vi "DebianFile.vi"(8 "error in (no error)":errorcluster, 11 "Package Builder in":refnum<class "Package Builder.lvclass">) -> (0 "error out":errorcluster, 3 "Package Builder out":refnum<class "Package Builder.lvclass">)   [LabVIEW 2020, in "Package Builder.lvclass"]
uses:
  Package Builder.lvclass
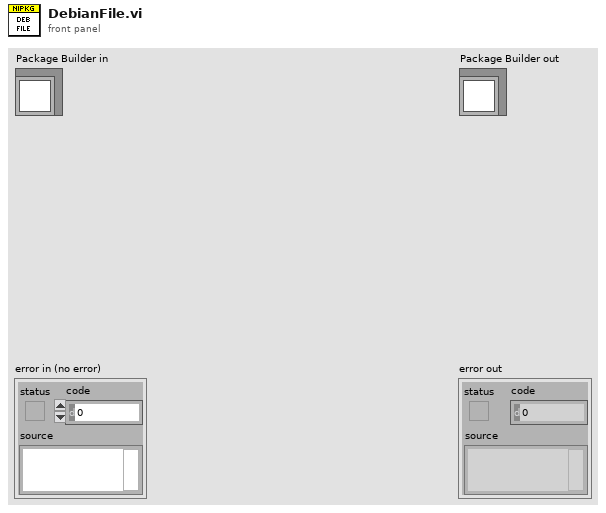
[diagram p1: front panel]
types:
  T1 = enum16{"open", "replace", "create", "open or create", "replace or create", "replace or create with confirmation"}
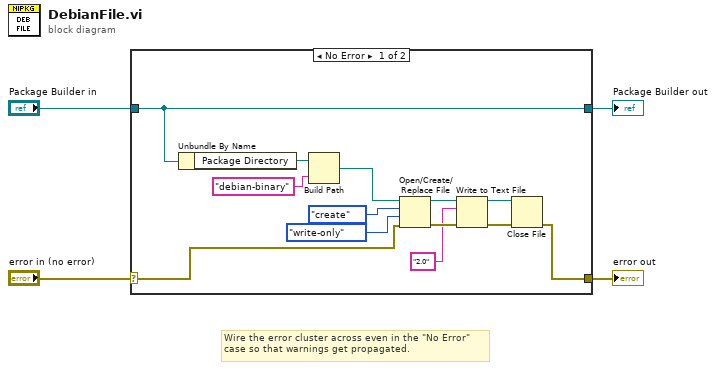
[diagram p0: block diagram]
diagram:
  # "Wire the error cluster across even in the \"No Error\"\ncase so that warnings get propagated."
  n1 = case shown="No Error" "error in (no error)" {
    selector: "error in (no error)" -> [w6 w19]
    tunnel: [w5 w19] -> w3
    tunnel: [w8 w18] -> w1
    tunnel: "Package Builder in" -> [w8 w18]
    frame No Error {
      n2 = Unbundle By Name(w8) -> ("Package Directory"=w7:path)
      n3 = Build Path(base path=w7, name or relative path="debian-binary" ("time format string (%c)")) -> (appended path=w10:path)
      n4 = Open/Create/Replace File(file path (use dialog)=w10, error in=w6, operation (0:open)=T1."create", access (0:read/write)=enum16{"read/write", "read-only", "write-only"}."write-only") -> (refnum out=w15:refnum<file>, error out=w14:errorcluster)  [unwired: 2 in, 1 out]
      n5 = Write to Text File(file (use dialog)=w15, text="2.0", error in=w14) -> (refnum out=w16:refnum<file>, error out=w17:errorcluster)  [unwired: 1 in, 1 out]
      n6 = Close File(refnum=w16, error in=w17) -> (error out=w5:errorcluster)  [unwired: 1 out]
    }
    frame Error {
    }
  }
  "error out" <- w3
  "Package Builder out" <- w1
